vi "SysGlbs.vi"() -> ()   [LabVIEW 2011]
panel:
  in  "Ganzilla?":bool
  in  "DNet?":bool
  in  "CTC_Auto?":bool
  in  "Dual O-Ring":T1
  in  "Shrouds":T2={"Alk Inj"=[52, 53, 54], "Alk2 Inj"=[], "Hyd Inj"=[], "H2 Shroud"=[20, 21], "H2 Purge"=[]}
  in  "Facility Outputs":T3={"Green"=124, "Amber"=127, "Red"=126, " Blue"=128, "Audible Alarm"=125, "Toxic Alarm"=0}
  in  "ExtCtrl":bool
  in  "Shutter":cluster{"Din":i32, "Dout":i32}={"Din"=125, "Dout"=125}
  in  "Epison":T4={"MFC#"=[2], "EPS#"=[35], "Epison?"=TRUE}
  in  "N2 Standby":T5={"Valves"=[48, 49, 50, 51, 52, 53], "Analog"=[40, 41, 42, 43, 44, 45], "A_Value%"=[1.0, 1.0, 1.0, 1.0, 0.0, 1.0, 1.0, 1.0, 0.5], "Bypass"=FALSE, "Bypass Valve"=0, "Pumps"=[1, 1, 1, 1, 0, 1, 1, 1, 0], "Inj Vent"=[40, 41, 42, 43, 44, 45]} {"A_Value%" format="%.2f"}
  in  "DIdleN2":bool[](array[boolean])
  in  "DIdleH":bool[](array[boolean])
  in  "DIdler":bool[](array[boolean])
  in  "DIdle":bool[](array[boolean])
  in  "AIdleN2":dbl[](array[numeric]) format="%.2f"
  in  "AIdleH":dbl[](array[numeric]) format="%.2f"
  in  "AIdler":dbl[](array[numeric]) format="%.2f"
  in  "AIdle":dbl[](array[numeric]) format="%.2f"
  in  "Gold?":bool
  in  "constants":T6 {"LL Fill Press" format="%.2f"; "PP Cycles" format="%.2f"; "GV Interlock" format="%.2f"; "LPC Fill Flow" format="%.2f"; "LPC Fill Rate" format="%.2f"; "LL Fill Rate" format="%.2f"; "GC Ramp Rate" format="%.2f"; "LL Fill Flow" format="%.2f"; "Ring On Press" format="%.2f"; "Shutdown Press" format="%.2f"; "GC Idle Switch" format="%.2f"; "LL Switch Press" format="%.2f"; "AtomPress" format="%.2f"}
  in  "Convectron":i32[](array[numeric])=[55]
  in  "Ion":i32[](array[numeric])=[54]
  in  "notifier":T7
  in  "ROnly":bool[](array[boolean])=[FALSE, FALSE, FALSE, FALSE, FALSE, FALSE, FALSE, FALSE, FALSE, FALSE, FALSE, FALSE, FALSE, FALSE, FALSE, FALSE, FALSE, FALSE, FALSE, FALSE, FALSE, FALSE, FALSE, FALSE, FALSE, FALSE, FALSE, FALSE, FALSE, FALSE, FALSE, FALSE, FALSE, FALSE, FALSE, TRUE, TRUE, FALSE, TRUE, FALSE, FALSE, FALSE, FALSE, FALSE, FALSE, FALSE, FALSE, FALSE, FALSE, FALSE, FALSE, FALSE, FALSE, FALSE, FALSE, FALSE, FALSE, FALSE, FALSE, FALSE, TRUE, TRUE, TRUE, TRUE, TRUE, TRUE, FALSE, FALSE, FALSE, TRUE, TRUE, TRUE, FALSE, FALSE, FALSE, FALSE, FALSE, FALSE, FALSE, FALSE, FALSE]
  in  "Full":i32[](array[numeric])=[55]
  in  "Pirani":i32[](array[numeric])=[54]
  in  "Purge_Line":T8={"Valves"=[48, 49, 50, 51, 52, 53], "Analog"=[40, 41, 42, 43, 44, 45], "A_Value%"=[1.0, 1.0, 1.0, 1.0, 0.0, 1.0, 1.0, 1.0, 0.5]} {"A_Value%" format="%.2f"}
  in  "Digital #":u32=128
  in  "Analog #":u32=72
  in  "get?":bool
  in  "Set Chg":bool
  in  "mV high":i32[](array[numeric])=[5000, 5000, 5000, 5000, 5000, 5000, 5000, 5000, 5000, 5000, 10000, 10000, 10000, 10000, 10000, 10000, 10000, 10000, 10000, 5000, 5000, 10000, 5000, 5000, 10000, 10000, 10000, 10000, 5000, 5000, 5000, 5000, 10000, 5000, 5000, 10000, 10000, 10000, 10000, 10000, 5000, 5000, 5000, 5000, 5000, 5000, 5000, 5000, 5000, 5000, 5000, 5000, 5000, 5000, 5000, 5000, 5000, 5000, 5000, 5000, 0, 0, 0, 0, 0, 0, 10000, 5000, 5000, 5000, 10000, 10000]
  in  "mV low":i32[](array[numeric])=[0, 0, 0, 0, 0, 0, 0, 0, 0, 0, 0, 0, 0, 0, 0, 0, 0, 0, 0, 0, 0, 0, 0, 0, 0, 0, 0, 0, 0, 0, 0, 0, 0, 0, 0, 0, 0, 0, 0, 0, 0, 0, 0, 0, 0, 0, 0, 0, 0, 0, 0, 0, 0, 0, 0, 0, 0, 0, 0, 0, 0, 0, 0, 0, 0, 0, 0, 0, 0, 0, 0, 0]
  in  "Offset":i32[](array[numeric])=[0, 0, 0, 0, 0, 0, 0, 0, 0, 0, 0, 0, 0, 0, 0, 0, 0, 0, 0, 0, 0, 0, 0, 0, 0, -100, 0, -100, 0, 0, 0, 0, 0, 0, 0, 0, 0, 0, 0, 0, 0, 0, 0, 0, 0, 0, 0, 0, 0, 0, 0, 0, 0, 0, 0, 0, 0, 0, 0, 0, 0, 0, 0, 0, 0, 0, 0, 0, 0, 0, 450, 450]
  in  "Analog List":string[](array[string])=["MFC1", "MFC2", "MFC3", "MFC4", "MFC5", "MFC6", "MFC7", "MFC8", "MFC9", "MFC10", "Press11", "Press12", "Press13", "Press14", "Press15", "Press16", "Press17", "Press18", "Press19", "MFC20", "MFC21", "Press22", "MFC23", "MFC24", "Press25", "Press26", "Press27", "Press28", "MFC29", "MFC30", "MFC31", "MFC32", "Motor33", "Temp34", "Temp35", "Press36", "Press37", "Press38", "Press39", "Press40", "MFC41", "MFC42", "MFC43", "MFC44", "MFC45", "MFC46", "MFC47", "MFC48", "MFC49", "MFC50", "MFC51", "MFC52", "MFC53", "MFC54", "MFC55", "MFC56", "MFC57", "MFC58", "MFC59", "MFC60", "Epison61", "Epison62", "Epison63", "Epison64", "Epison65", "Epison66", "Motor67", "Temp68", "Temp69", "Temp70", "Temp71", "Temp72"]
  in  "Control Names":string[](array[string])=["DEZn", "TMIn #1", "TMIn #2", "TEG", "TMG", "TMAl", "Fe", "TBP", "TBA", "Spare", "TMIn1 Press", "TMIn2 Press", "TEG Press", "TMG Press", "TMAl Press", "Fe Press", "TBP Press", "TBA Press", "Spare Press", "DEZn DD", "DEZn w/DD", "DEZn Press", "N2 Purge2", "N2 Purge", "Alk Inj Press", "Alk Diff Press", "Hyd Inj Press", "Hyd Diff Press", "Alk Inj Push", "Alk Vent Push", "Hyd Inj Push", "Hyd Vent Push", "Motor", "T/C Out", "T/C In", "LL Press2", "LL Press", "GC Press", "Vac Press", "GC Press2", "AsH3#1", "AsH3 #2", "PH3", "Hyd Spare1", "Hyd Spare2", "Hyd Spare3", "H2 Shroud2", "H2 Shroud", "Hyd Inj Out", "Hyd Inj Mid", "Hyd Inj In", "Alk Inj Out", "Alk Inj Mid", "Alk Inj In", "Hyd Inj Out2", "Hyd Inj Mid2", "Hyd Inj In2", "Alk Inj Out2", "Alk Inj Mid2", "Alk Inj In2", "Epison #1", "Epison #2", "Epi/Min1", "Epi/Min2", "Epi/Min3", "Epi/min4", "Motor2", "T/C Out2", "T/C In2", "PD Cell", "Sub Pyro1", "Sub Pyro2"]
  in  "Units":u8[](array[numeric])=[1, 1, 1, 1, 1, 1, 1, 1, 1, 1, 1, 1, 1, 1, 1, 1, 1, 1, 1, 1, 1, 1, 10, 10, 1, 1, 1, 1, 1, 1, 1, 1, 1, 1, 1, 1, 1, 1, 1, 1, 1, 1, 1, 1, 1, 1, 10, 10, 1, 1, 1, 1, 1, 1, 1, 1, 1, 1, 1, 1, 1, 1, 1, 1, 1, 1, 1, 1, 1, 1, 1, 1]
  in  "Scale":i32[](array[numeric])=[200, 1000, 500, 200, 100, 100, 100, 500, 500, 500, 1000, 1000, 1000, 1000, 1000, 1000, 1000, 1000, 1000, 2000, 200, 1000, 1000, 1000, 1000, 100, 1000, 100, 5000, 5000, 5000, 5000, 1185, 1500, 1500, 1000, 1000, 1000, 10000, 1000, 20, 500, 1000, 200, 200, 50, 5000, 5000, 1000, 500, 250, 1000, 500, 250, 1000, 500, 250, 1000, 500, 250, 0, 0, 0, 0, 0, 0, 1185, 1500, 1500, 500, 1500, 1500]
  in  "Inject":T9={"Alk Inj"=29, "Alk Inj Press"=25, "Alk vent"=30, "Alk vent Press"=26, "Hyd Inj"=31, "Hyd Inj Press"=27, "Hyd vent"=32, "Hyd vent Press"=28, "Spare Inj"=31, "Spare Inj  Press"=32, "Spare Vent"=28, "Spare Vent Press"=31}
  in  "Title":string="ORTEL SYSTEM THREE"
  in  "SysVal":i16[][](array[numeric])=[[1, 3, 5, 7, 9, 11, 13, 15, 17, 19, 3, 5, 7, 9, 11, 13, 15, 17, 19, 1, 1, 1, 0, 0, 0, 0, 0, 0, 0, 0, 0, 0, 0, 0, 0, 0, 0, 0, 0, 0, 49, 50, 51, 52, 53, 0, 54, 0, 0, 0, 0, 0, 0, 0, 0, 0], [2, 4, 6, 8, 10, 12, 14, 16, 18, 20, 4, 6, 8, 10, 12, 14, 16, 18, 20, 2, 2, 2, 0, 0, 0, 0, 0, 0, 0, 0, 0, 0, 0, 0, 0, 0, 0, 0, 0, 0, 55, 56, 57, 58, 59, 0, 60, 0, 0, 0, 0, 0, 0, 0, 0, 0], [47, 43, 41, 39, 37, 35, 25, 67, 65, 33, 43, 41, 39, 37, 35, 25, 67, 65, 33, 47, 47, 47, 0, 0, 0, 0, 0, 0, 0, 0, 0, 0, 0, 0, 0, 0, 0, 0, 0, 0, 79, 77, 75, 73, 71, 0, 45, 0, 0, 0, 0, 0, 0, 0, 0, 0], [48, 44, 42, 40, 38, 36, 26, 0, 66, 34, 44, 42, 40, 38, 36, 26, 0, 66, 34, 48, 48, 48, 0, 0, 0, 0, 0, 0, 0, 0, 0, 0, 0, 0, 0, 0, 0, 0, 0, 0, 80, 78, 76, 74, 72, 0, 46, 0, 0, 0, 0, 0, 0, 0, 0, 0], [81, 0, 0, 0, 0, 0, 87, 0, 0, 0, 0, 0, 0, 0, 0, 87, 0, 0, 0, 81, 81, 81, 0, 0, 0, 0, 0, 0, 0, 0, 0, 0, 0, 0, 0, 0, 0, 0, 0, 0, 0, 0, 0, 0, 0, 0, 0, 0, 0, 0, 0, 0, 0, 0, 0, 0], [0, 0, 0, 0, 0, 0, 88, 0, 0, 0, 0, 0, 0, 0, 0, 88, 0, 0, 0, 0, 0, 0, 0, 0, 0, 0, 0, 0, 0, 0, 0, 0, 0, 0, 0, 0, 0, 0, 0, 0, 0, 0, 0, 0, 0, 0, 0, 0, 0, 0, 0, 0, 0, 0, 0, 0], [0, 0, 0, 0, 0, 0, 0, 0, 0, 0, 0, 0, 0, 0, 0, 0, 0, 0, 0, 0, 0, 0, 0, 0, 0, 0, 0, 0, 0, 0, 0, 0, 0, 0, 0, 0, 0, 0, 0, 0, 0, 0, 0, 0, 0, 0, 0, 0, 0, 0, 0, 0, 0, 0, 0, 0], [0, 0, 0, 0, 0, 0, 0, 0, 0, 0, 0, 0, 0, 0, 0, 0, 0, 0, 0, 0, 0, 0, 0, 0, 0, 0, 0, 0, 0, 0, 0, 0, 0, 0, 0, 0, 0, 0, 0, 0, 0, 0, 0, 0, 0, 0, 0, 0, 0, 0, 0, 0, 0, 0, 0, 0], [0, 0, 0, 0, 0, 0, 0, 0, 0, 0, 0, 0, 0, 0, 0, 0, 0, 0, 0, 0, 0, 0, 0, 0, 0, 0, 0, 0, 0, 0, 0, 0, 0, 0, 0, 0, 0, 0, 0, 0, 0, 0, 0, 0, 0, 0, 0, 0, 0, 0, 0, 0, 0, 0, 0, 0], [0, 0, 0, 0, 0, 0, 0, 0, 0, 0, 0, 0, 0, 0, 0, 0, 0, 0, 0, 0, 0, 0, 0, 0, 0, 0, 0, 0, 0, 0, 0, 0, 0, 0, 0, 0, 0, 0, 0, 0, 0, 0, 0, 0, 0, 0, 0, 0, 0, 0, 0, 0, 0, 0, 0, 0], [0, 0, 0, 0, 0, 0, 0, 0, 0, 0, 0, 0, 0, 0, 0, 0, 0, 0, 0, 0, 0, 0, 0, 0, 0, 0, 0, 0, 0, 0, 0, 0, 0, 0, 0, 0, 0, 0, 0, 0, 0, 0, 0, 0, 0, 0, 0, 0, 0, 0, 0, 0, 0, 0, 0, 0], [0, 0, 0, 0, 0, 0, 0, 0, 0, 0, 0, 0, 0, 0, 0, 0, 0, 0, 0, 0, 0, 0, 0, 0, 0, 0, 0, 0, 0, 0, 0, 0, 0, 0, 0, 0, 0, 0, 0, 0, 0, 0, 0, 0, 0, 0, 0, 0, 0, 0, 0, 0, 0, 0, 0, 0], [0, 0, 0, 0, 0, 0, 0, 0, 0, 0, 0, 0, 0, 0, 0, 0, 0, 0, 0, 0, 0, 0, 0, 0, 0, 0, 0, 0, 0, 0, 0, 0, 0, 0, 0, 0, 0, 0, 0, 0, 0, 0, 0, 0, 0, 0, 0, 0, 0, 0, 0, 0, 0, 0, 0, 0], [0, 0, 0, 0, 0, 0, 0, 0, 0, 0, 0, 0, 0, 0, 0, 0, 0, 0, 0, 0, 0, 0, 0, 0, 0, 0, 0, 0, 0, 0, 0, 0, 0, 0, 0, 0, 0, 0, 0, 0, 0, 0, 0, 0, 0, 0, 0, 0, 0, 0, 0, 0, 0, 0, 0, 0], [0, 0, 0, 0, 0, 0, 0, 0, 0, 0, 0, 0, 0, 0, 0, 0, 0, 0, 0, 0, 0, 0, 0, 0, 0, 0, 0, 0, 0, 0, 0, 0, 0, 0, 0, 0, 0, 0, 0, 0, 0, 0, 0, 0, 0, 0, 0, 0, 0, 0, 0, 0, 0, 0, 0, 0], [0, 0, 0, 0, 0, 0, 0, 0, 0, 0, 0, 0, 0, 0, 0, 0, 0, 0, 0, 0, 0, 0, 0, 0, 0, 0, 0, 0, 0, 0, 0, 0, 0, 0, 0, 0, 0, 0, 0, 0, 0, 0, 0, 0, 0, 0, 0, 0, 0, 0, 0, 0, 0, 0, 0, 0], [0, 0, 0, 0, 0, 0, 0, 0, 0, 0, 0, 0, 0, 0, 0, 0, 0, 0, 0, 0, 0, 0, 0, 0, 0, 0, 0, 0, 0, 0, 0, 0, 0, 0, 0, 0, 0, 0, 0, 0, 0, 0, 0, 0, 0, 0, 0, 0, 0, 0, 0, 0, 0, 0, 0, 0], [0, 0, 0, 0, 0, 0, 0, 0, 0, 0, 0, 0, 0, 0, 0, 0, 0, 0, 0, 0, 0, 0, 0, 0, 0, 0, 0, 0, 0, 0, 0, 0, 0, 0, 0, 0, 0, 0, 0, 0, 0, 0, 0, 0, 0, 0, 0, 0, 0, 0, 0, 0, 0, 0, 0, 0], [0, 0, 0, 0, 0, 0, 0, 0, 0, 0, 0, 0, 0, 0, 0, 0, 0, 0, 0, 0, 0, 0, 0, 0, 0, 0, 0, 0, 0, 0, 0, 0, 0, 0, 0, 0, 0, 0, 0, 0, 0, 0, 0, 0, 0, 0, 0, 0, 0, 0, 0, 0, 0, 0, 0, 0], [0, 0, 0, 0, 0, 0, 0, 0, 0, 0, 0, 0, 0, 0, 0, 0, 0, 0, 0, 0, 0, 0, 0, 0, 0, 0, 0, 0, 0, 0, 0, 0, 0, 0, 0, 0, 0, 0, 0, 0, 0, 0, 0, 0, 0, 0, 0, 0, 0, 0, 0, 0, 0, 0, 0, 0], [0, 0, 0, 0, 0, 0, 0, 0, 0, 0, 0, 0, 0, 0, 0, 0, 0, 0, 0, 0, 0, 0, 0, 0, 0, 0, 0, 0, 0, 0, 0, 0, 0, 0, 0, 0, 0, 0, 0, 0, 0, 0, 0, 0, 0, 0, 0, 0, 0, 0, 0, 0, 0, 0, 0, 0], [0, 0, 0, 0, 0, 0, 0, 0, 0, 0, 0, 0, 0, 0, 0, 0, 0, 0, 0, 0, 0, 0, 0, 0, 0, 0, 0, 0, 0, 0, 0, 0, 0, 0, 0, 0, 0, 0, 0, 0, 0, 0, 0, 0, 0, 0, 0, 0, 0, 0, 0, 0, 0, 0, 0, 0], [0, 0, 0, 0, 0, 0, 0, 0, 0, 0, 0, 0, 0, 0, 0, 0, 0, 0, 0, 0, 0, 0, 0, 0, 0, 0, 0, 0, 0, 0, 0, 0, 0, 0, 0, 0, 0, 0, 0, 0, 0, 0, 0, 0, 0, 0, 0, 0, 0, 0, 0, 0, 0, 0, 0, 0], [0, 0, 0, 0, 0, 0, 0, 0, 0, 0, 0, 0, 0, 0, 0, 0, 0, 0, 0, 0, 0, 0, 0, 0, 0, 0, 0, 0, 0, 0, 0, 0, 0, 0, 0, 0, 0, 0, 0, 0, 0, 0, 0, 0, 0, 0, 0, 0, 0, 0, 0, 0, 0, 0, 0, 0], [0, 0, 0, 0, 0, 0, 0, 0, 0, 0, 0, 0, 0, 0, 0, 0, 0, 0, 0, 0, 0, 0, 0, 0, 0, 0, 0, 0, 0, 0, 0, 0, 0, 0, 0, 0, 0, 0, 0, 0, 0, 0, 0, 0, 0, 0, 0, 0, 0, 0, 0, 0, 0, 0, 0, 0], [0, 0, 0, 0, 0, 0, 0, 0, 0, 0, 0, 0, 0, 0, 0, 0, 0, 0, 0, 0, 0, 0, 0, 0, 0, 0, 0, 0, 0, 0, 0, 0, 0, 0, 0, 0, 0, 0, 0, 0, 0, 0, 0, 0, 0, 0, 0, 0, 0, 0, 0, 0, 0, 0, 0, 0], [0, 0, 0, 0, 0, 0, 0, 0, 0, 0, 0, 0, 0, 0, 0, 0, 0, 0, 0, 0, 0, 0, 0, 0, 0, 0, 0, 0, 0, 0, 0, 0, 0, 0, 0, 0, 0, 0, 0, 0, 0, 0, 0, 0, 0, 0, 0, 0, 0, 0, 0, 0, 0, 0, 0, 0], [0, 0, 0, 0, 0, 0, 0, 0, 0, 0, 0, 0, 0, 0, 0, 0, 0, 0, 0, 0, 0, 0, 0, 0, 0, 0, 0, 0, 0, 0, 0, 0, 0, 0, 0, 0, 0, 0, 0, 0, 0, 0, 0, 0, 0, 0, 0, 0, 0, 0, 0, 0, 0, 0, 0, 0], [0, 0, 0, 0, 0, 0, 0, 0, 0, 0, 0, 0, 0, 0, 0, 0, 0, 0, 0, 0, 0, 0, 0, 0, 0, 0, 0, 0, 0, 0, 0, 0, 0, 0, 0, 0, 0, 0, 0, 0, 0, 0, 0, 0, 0, 0, 0, 0, 0, 0, 0, 0, 0, 0, 0, 0], [0, 0, 0, 0, 0, 0, 0, 0, 0, 0, 0, 0, 0, 0, 0, 0, 0, 0, 0, 0, 0, 0, 0, 0, 0, 0, 0, 0, 0, 0, 0, 0, 0, 0, 0, 0, 0, 0, 0, 0, 0, 0, 0, 0, 0, 0, 0, 0, 0, 0, 0, 0, 0, 0, 0, 0], [0, 0, 0, 0, 0, 0, 0, 0, 0, 0, 0, 0, 0, 0, 0, 0, 0, 0, 0, 0, 0, 0, 0, 0, 0, 0, 0, 0, 0, 0, 0, 0, 0, 0, 0, 0, 0, 0, 0, 0, 0, 0, 0, 0, 0, 0, 0, 0, 0, 0, 0, 0, 0, 0, 0, 0], [0, 0, 0, 0, 0, 0, 0, 0, 0, 0, 0, 0, 0, 0, 0, 0, 0, 0, 0, 0, 0, 0, 0, 0, 0, 0, 0, 0, 0, 0, 0, 0, 0, 0, 0, 0, 0, 0, 0, 0, 0, 0, 0, 0, 0, 0, 0, 0, 0, 0, 0, 0, 0, 0, 0, 0], [0, 0, 0, 0, 0, 0, 0, 0, 0, 0, 0, 0, 0, 0, 0, 0, 0, 0, 0, 0, 0, 0, 0, 0, 0, 0, 0, 0, 0, 0, 0, 0, 0, 0, 0, 0, 0, 0, 0, 0, 0, 0, 0, 0, 0, 0, 0, 0, 0, 0, 0, 0, 0, 0, 0, 0], [0, 0, 0, 0, 0, 0, 0, 0, 0, 0, 0, 0, 0, 0, 0, 0, 0, 0, 0, 0, 0, 0, 0, 0, 0, 0, 0, 0, 0, 0, 0, 0, 0, 0, 0, 0, 0, 0, 0, 0, 0, 0, 0, 0, 0, 0, 0, 0, 0, 0, 0, 0, 0, 0, 0, 0], [0, 0, 0, 0, 0, 0, 0, 0, 0, 0, 0, 0, 0, 0, 0, 0, 0, 0, 0, 0, 0, 0, 0, 0, 0, 0, 0, 0, 0, 0, 0, 0, 0, 0, 0, 0, 0, 0, 0, 0, 0, 0, 0, 0, 0, 0, 0, 0, 0, 0, 0, 0, 0, 0, 0, 0], [0, 0, 0, 0, 0, 0, 0, 0, 0, 0, 0, 0, 0, 0, 0, 0, 0, 0, 0, 0, 0, 0, 0, 0, 0, 0, 0, 0, 0, 0, 0, 0, 0, 0, 0, 0, 0, 0, 0, 0, 0, 0, 0, 0, 0, 0, 0, 0, 0, 0, 0, 0, 0, 0, 0, 0], [0, 0, 0, 0, 0, 0, 0, 0, 0, 0, 0, 0, 0, 0, 0, 0, 0, 0, 0, 0, 0, 0, 0, 0, 0, 0, 0, 0, 0, 0, 0, 0, 0, 0, 0, 0, 0, 0, 0, 0, 0, 0, 0, 0, 0, 0, 0, 0, 0, 0, 0, 0, 0, 0, 0, 0], [0, 0, 0, 0, 0, 0, 0, 0, 0, 0, 0, 0, 0, 0, 0, 0, 0, 0, 0, 0, 0, 0, 0, 0, 0, 0, 0, 0, 0, 0, 0, 0, 0, 0, 0, 0, 0, 0, 0, 0, 0, 0, 0, 0, 0, 0, 0, 0, 0, 0, 0, 0, 0, 0, 0, 0], [0, 0, 0, 0, 0, 0, 0, 0, 0, 0, 0, 0, 0, 0, 0, 0, 0, 0, 0, 0, 0, 0, 0, 0, 0, 0, 0, 0, 0, 0, 0, 0, 0, 0, 0, 0, 0, 0, 0, 0, 0, 0, 0, 0, 0, 0, 0, 0, 0, 0, 0, 0, 0, 0, 0, 0], [0, 0, 0, 0, 0, 0, 0, 0, 0, 0, 0, 0, 0, 0, 0, 0, 0, 0, 0, 0, 0, 0, 0, 0, 0, 0, 0, 0, 0, 0, 0, 0, 0, 0, 0, 0, 0, 0, 0, 0, 0, 0, 0, 0, 0, 0, 0, 0, 0, 0, 0, 0, 0, 0, 0, 0], [0, 0, 0, 0, 0, 0, 0, 0, 0, 0, 0, 0, 0, 0, 0, 0, 0, 0, 0, 0, 0, 0, 0, 0, 0, 0, 0, 0, 0, 0, 0, 0, 0, 0, 0, 0, 0, 0, 0, 0, 0, 0, 0, 0, 0, 0, 0, 0, 0, 0, 0, 0, 0, 0, 0, 0], [0, 0, 0, 0, 0, 0, 0, 0, 0, 0, 0, 0, 0, 0, 0, 0, 0, 0, 0, 0, 0, 0, 0, 0, 0, 0, 0, 0, 0, 0, 0, 0, 0, 0, 0, 0, 0, 0, 0, 0, 0, 0, 0, 0, 0, 0, 0, 0, 0, 0, 0, 0, 0, 0, 0, 0], [0, 0, 0, 0, 0, 0, 0, 0, 0, 0, 0, 0, 0, 0, 0, 0, 0, 0, 0, 0, 0, 0, 0, 0, 0, 0, 0, 0, 0, 0, 0, 0, 0, 0, 0, 0, 0, 0, 0, 0, 0, 0, 0, 0, 0, 0, 0, 0, 0, 0, 0, 0, 0, 0, 0, 0], [0, 0, 0, 0, 0, 0, 0, 0, 0, 0, 0, 0, 0, 0, 0, 0, 0, 0, 0, 0, 0, 0, 0, 0, 0, 0, 0, 0, 0, 0, 0, 0, 0, 0, 0, 0, 0, 0, 0, 0, 0, 0, 0, 0, 0, 0, 0, 0, 0, 0, 0, 0, 0, 0, 0, 0], [0, 0, 0, 0, 0, 0, 0, 0, 0, 0, 0, 0, 0, 0, 0, 0, 0, 0, 0, 0, 0, 0, 0, 0, 0, 0, 0, 0, 0, 0, 0, 0, 0, 0, 0, 0, 0, 0, 0, 0, 0, 0, 0, 0, 0, 0, 0, 0, 0, 0, 0, 0, 0, 0, 0, 0], [0, 0, 0, 0, 0, 0, 0, 0, 0, 0, 0, 0, 0, 0, 0, 0, 0, 0, 0, 0, 0, 0, 0, 0, 0, 0, 0, 0, 0, 0, 0, 0, 0, 0, 0, 0, 0, 0, 0, 0, 0, 0, 0, 0, 0, 0, 0, 0, 0, 0, 0, 0, 0, 0, 0, 0], [0, 0, 0, 0, 0, 0, 0, 0, 0, 0, 0, 0, 0, 0, 0, 0, 0, 0, 0, 0, 0, 0, 0, 0, 0, 0, 0, 0, 0, 0, 0, 0, 0, 0, 0, 0, 0, 0, 0, 0, 0, 0, 0, 0, 0, 0, 0, 0, 0, 0, 0, 0, 0, 0, 0, 0]]
  in  "Alk/Hyd":T10={"Alk Index"=[1, 2, 3, 4, 5, 6, 7, 8, 9], "Alk Grow"=[47, 43, 41, 39, 37, 35, 25, 67, 65, 73, 71, 69, 61, 63, 65, 67, 59, 49], "Alk Vent"=[2, 4, 6, 8, 10, 12, 14, 16, 18], "Alk Press"=[22, 11, 12, 13, 14, 15, 16, 17, 18], "Hyd Index"=[41, 42, 43, 44, 45, 46], "Hyd Grow"=[79, 77, 75, 73, 71, 45], "Hyd Vent"=[49, 50, 51, 52, 53, 54], "Hyd Press"=[0, 0, 0, 0, 0, 0], "Alk Primary"=[], "Hyd Primary"=[]}
  in  "Ch Assign":T11={"Press"=[9, 10, 11, 12, 13, 14, 15, 16, 17], "PD_cell"={"H2_cell"=22, "H2_line"=21, "horn"=112, "light"=113, "temp"=69, "PD_cell?"=TRUE, "Temp Set"=0, "N2_in"=20, "N2_line"=0}, "RampDn"=[32], "GV/LL"={"LL Door"=96, "GV Up"=98, "GV Low"=99, "GV _LIn"=18, "Fork"=19, "GV_UIn"=17, "GC Press"=37, "LL Press"=36, "MDA_LL"=[38], "Motor"=19, "EQ Valve"=99, "LL Active"=19}, "GC_Pump"={"LL_Vac"=100, "GC_Vac"=102, "Bypass"=104, "Rough"=105, "Isolat"=110, "LL_MDA"=[101], "Vac_Press"=38, "TGV"=102}, "N2 Purge"={"N2_LL"=45, "MFC"=23}, "RampRate"=[20.0], "GC_Vac"={"D_Vac-"=[38, 43, 44, 45, 46, 47, 81, 82, 83, 104, 110], "D_Vac+"=[], "A_Vac"=[24, 26, 37, 40, 41, 42, 44, 50, 51, 64, 65, 66, 67, 68, 69, 70, 71], "D_Open+"=[104], "D_Open-"=[105, 110], "A_Open"=[24, 26, 40, 41, 42, 50, 51, 64, 65, 66, 67, 68, 69, 70, 71]}, "Toxic"=[48, 49, 50], "Indicators"=[108, 114], "LL Routine"={"D Open"=[39], "D Close"=[], "Timeout(ms)"=150000}, "Temperature"=[], "EBARA Pump"={"EBARA_Din"={"Main Status"=43, "Booster Status"=0, "Indicator"=114, "N2 Isolat"=93}, "EBARA_N2"=[6]}} {"RampRate" format="%.2f"}
  # "Analog Settings"
  # "Idles"
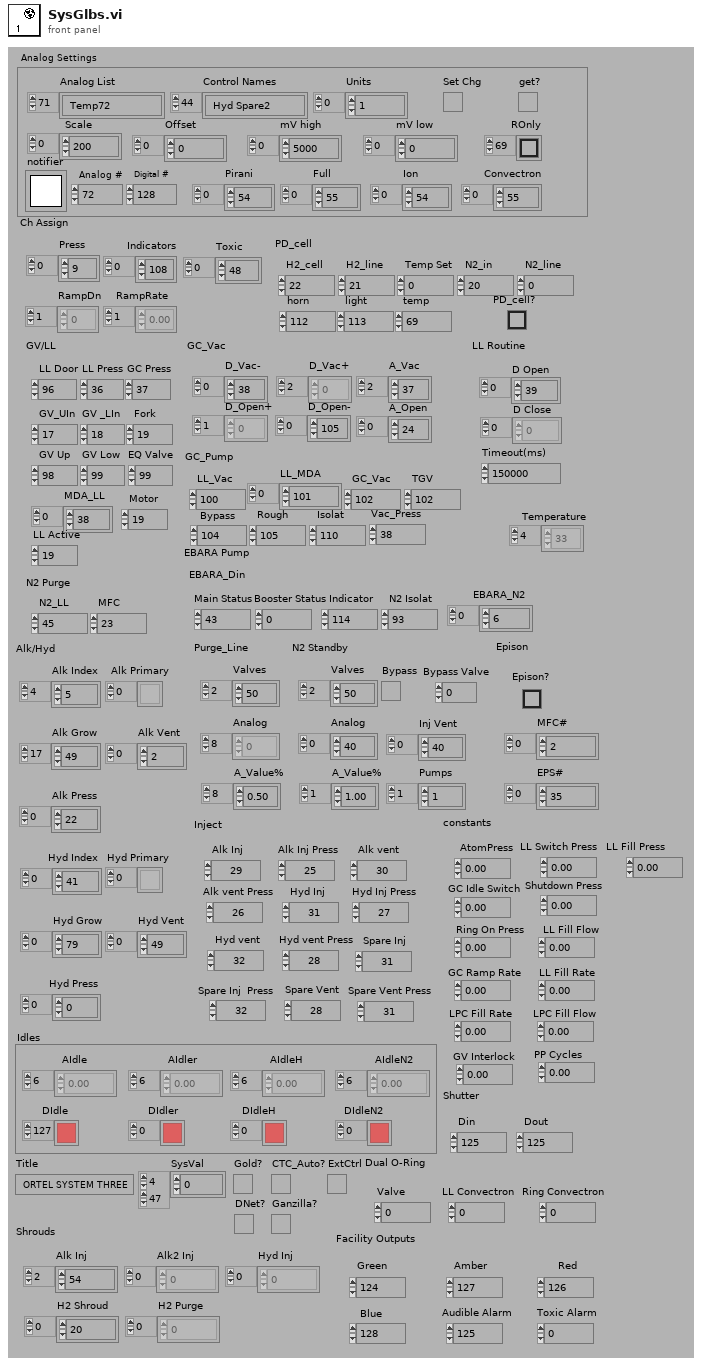
[diagram p1: front panel]
types:
  T1 = cluster{"Valve":i32, "LL Convectron":i32, "Ring Convectron":i32}
  T2 = cluster{"Alk Inj":i32[], "Alk2 Inj":i32[], "Hyd Inj":i32[], "H2 Shroud":i32[], "H2 Purge":i32[]}
  T3 = cluster{"Green":u16, "Amber":u16, "Red":u16, " Blue":u16, "Audible Alarm":u16, "Toxic Alarm":u16}
  T4 = cluster{"MFC#":u8[], "EPS#":u8[], "Epison?":bool}
  T5 = cluster{"Valves":u16[], "Analog":u16[], "A_Value%":dbl[], "Bypass":bool, "Bypass Valve":u16, "Pumps":i32[], "Inj Vent":u16[]}
  T6 = cluster{"AtomPress":dbl, "LL Switch Press":dbl, "GC Idle Switch":dbl, "Shutdown Press":dbl, "Ring On Press":dbl, "LL Fill Flow":dbl, "GC Ramp Rate":dbl, "LL Fill Rate":dbl, "LPC Fill Rate":dbl, "LPC Fill Flow":dbl, "GV Interlock":dbl, "PP Cycles":dbl, "LL Fill Press":dbl}
  T7 = typedef "Notifier RefNum" = refnum<k1>
  T8 = cluster{"Valves":u16[], "Analog":u16[], "A_Value%":dbl[]}
  T9 = cluster{"Alk Inj":u8, "Alk Inj Press":u8, "Alk vent":u8, "Alk vent Press":u8, "Hyd Inj":u8, "Hyd Inj Press":u8, "Hyd vent":u8, "Hyd vent Press":u8, "Spare Inj":u8, "Spare Inj  Press":u8, "Spare Vent":u8, "Spare Vent Press":u8}
  T10 = cluster{"Alk Index":u8[], "Alk Grow":u8[], "Alk Vent":u8[], "Alk Press":u8[], "Hyd Index":u8[], "Hyd Grow":u8[], "Hyd Vent":u8[], "Hyd Press":u8[], "Alk Primary":bool[], "Hyd Primary":bool[]}
  T11 = cluster{"Press":u8[], "PD_cell":cluster{"H2_cell":u8, "H2_line":u8, "horn":u8, "light":u8, "temp":u8, "PD_cell?":bool, "Temp Set":u16, "N2_in":u8, "N2_line":u8}, "RampDn":u8[], "GV/LL":cluster{"LL Door":u8, "GV Up":u8, "GV Low":u8, "GV _LIn":u8, "Fork":u8, "GV_UIn":u8, "GC Press":u8, "LL Press":u8, "MDA_LL":u8[], "Motor":u8, "EQ Valve":u8, "LL Active":u8}, "GC_Pump":cluster{"LL_Vac":u8, "GC_Vac":u8, "Bypass":u8, "Rough":u8, "Isolat":u8, "LL_MDA":u8[], "Vac_Press":u8, "TGV":u8}, "N2 Purge":cluster{"N2_LL":u8, "MFC":u8}, "RampRate":dbl[], "GC_Vac":cluster{"D_Vac-":u8[], "D_Vac+":u8[], "A_Vac":u8[], "D_Open+":u8[], "D_Open-":u8[], "A_Open":u8[]}, "Toxic":u8[], "Indicators":u8[], "LL Routine":cluster{"D Open":u8[], "D Close":u8[], "Timeout(ms)":u32}, "Temperature":u8[], "EBARA Pump":cluster{"EBARA_Din":cluster{"Main Status":u8, "Booster Status":u8, "Indicator":u8, "N2 Isolat":u8}, "EBARA_N2":u8[]}}
diagram:
